vi "HEWH Sampled Data String.vi"(8 "error in (no error)":errorcluster, 11 "UEF Calculated Values Output in":T1 {"Data Indexes"."15 sec after Draw Index" format="%#.2f"; "Data Indexes"."15 sec after Draw Timestamp" format="%#.2f"; "Data Indexes"."Test Start Timestamp" format="%.2f"; "Data Indexes"."Test End Timestamp" format="%.2f"; "Data Indexes"."T0 Timestamp" format="%.2f"; "Data Indexes"."Tsf Timestamp" format="%.2f"; "Data Indexes"."Tsu0 Timestamp" format="%.2f"; "Data Indexes"."Tmax1 Timestamp" format="%.2f"; "Data Indexes"."Draw Index Timestamp" format="%#.2f"; "Data Indexes"."Non-Draw Timestamp" format="%#.2f"; "Data Indexes"."Heating Timestamp" format="%#.2f"; "Data Indexes"."Start Energy (BTU-Gas)" format="%.6f"; "Data Indexes"."Start Watt Hours" format="%.6f"; "Static Data"."V - Volume of Wh (True)" format="%.5f"; "Static Data"."T-Ambinet Nominal (°F)" format="%.5f"; "Static Data"."T-Inlet Setpoint (°F)" format="%.5f"; "Static Data"."T-Wh Setpoint (°F)" format="%.5f"; "Sampled Data"."Qe (Wh)" format="%.5f"; "Sampled Data"."Tau stby2 (hr)" format="%.5f"; "Sampled Data"."Tastby2 (°F)" format="%.5f"; "Sampled Data"."Qf (BTU)" format="%.5f"; "Sampled Data"."Qe (BTU)" format="%.5f"; "Sampled Data"."Tmax1 (°F)" format="%.5f"; "Sampled Data"."T0 (°F)" format="%.5f"; "Sampled Data"."Qr (BTU)" format="%.5f"; "Sampled Data"."T 24(°F)" format="%.5f"; "Sampled Data"."T astby(°F)" format="%.5f"; "Sampled Data"."T tstby(°F)" format="%.5f"; "Sampled Data"."T su0(°F)" format="%.5f"; "Sampled Data"."T suf(°F)" format="%.5f"; "Sampled Data"."Tau stby_1 (hr)" format="%.5f"; "Sampled Data"."Qsuf (BTU)" format="%.5f"; "Sampled Data"."Qsu0 (BTU)" format="%.5f"; "Calculated Values"."Draw Bonus Volume (gal)" format="%.6f"; "Calculated Values"."Adjustment Factor" format="%.6f"; "Calculated Values"."T*avg_del(n-1)" format="%.6f"; "Calculated Values"."T*min(n-1)" format="%.6f"; "Calculated Values"."T*avg_del(n)" format="%.6f"; "Calculated Values"."Vn" format="%.6f"; "Calculated Values"."Qdm (BTU)" format="%.6f"; "Calculated Values"."QHWD (BTU)" format="%.6f"; "Calculated Values"."QHW (BTU)" format="%.6f"; "Calculated Values"."UEF" format="%.6f"; "Calculated Values"."QHW67 (BTU)" format="%.6f"; "Calculated Values"."Qda (BTU)" format="%.6f"; "Calculated Values"."Qd (BTU)" format="%.6f"; "Calculated Values"."Q (BTU)" format="%.6f"; "Calculated Values"."UA (BTU/(hr*F))" format="%.6f"; "Calculated Values"."Qhr (BTU/hr)" format="%.6f"; "Calculated Values"."Qstby (BTU)" format="%.6f"; "Calculated Values"."nu_r" format="%.6f"; "Calculated Values"."CpUEF (BTU/(lb*F))" format="%.6f"; "Calculated Values"."rho_nu (lb/gal)" format="%.6f"; "Calculated Values"."V1- Vol (Gal)" format="%.6f"; "Calculated Values"."M cluster mass removed (lb)" format="%.6f"; "Calculated Values"."Cp theoretical (BTU/(lbm °F))" format="%.6f"; "Calculated Values"."Tin1 - Mean Inlet 1st Cluster (°F)" format="%.6f"; "Calculated Values"."Tdel1-Mean Outlet 1st Cluster(°F)" format="%.6f"; "Calculated Values"."Cp 24 (BTU/(lb*F))" format="%.6f"; "Calculated Values"."Cp standby (BTU/(lb*F))" format="%.6f"; "Calculated Values"."Cp2 (BTU/(lb*F))" format="%.6f"; "Calculated Values"."Cp1 (BTU/(lb*F))" format="%.6f"; "Calculated Values"."rho 24 (lb/gal)" format="%.6f"; "Calculated Values"."rho standby (lb/gal)" format="%.6f"; "Calculated Values"."rho 2 (lb/gal)" format="%.6f"; "Calculated Values"."Density of cold water All (lbm/gal)" format="%#.3g"; "Calculated Values"."CpHW (BTU/(lbm °F))" format="%#.3g"; "Calculated Values"."Density of hot water All (lbm/gal)" format="%#.3g"; "Calculated Values"."Mass of water All (lbm)" format="%#.3f"}) -> (0 "error out":errorcluster, 3 "UEF Calculated Values Output out":T1 {"Data Indexes"."15 sec after Draw Index" format="%#.2f"; "Data Indexes"."15 sec after Draw Timestamp" format="%#.2f"; "Data Indexes"."Test Start Timestamp" format="%.2f"; "Data Indexes"."Test End Timestamp" format="%.2f"; "Data Indexes"."T0 Timestamp" format="%.2f"; "Data Indexes"."Tsf Timestamp" format="%.2f"; "Data Indexes"."Tsu0 Timestamp" format="%.2f"; "Data Indexes"."Tmax1 Timestamp" format="%.2f"; "Data Indexes"."Draw Index Timestamp" format="%#.2f"; "Data Indexes"."Non-Draw Timestamp" format="%#.2f"; "Data Indexes"."Heating Timestamp" format="%#.2f"; "Data Indexes"."Start Energy (BTU-Gas)" format="%.6f"; "Data Indexes"."Start Watt Hours" format="%.6f"; "Static Data"."V - Volume of Wh (True)" format="%.5f"; "Static Data"."T-Ambinet Nominal (°F)" format="%.5f"; "Static Data"."T-Inlet Setpoint (°F)" format="%.5f"; "Static Data"."T-Wh Setpoint (°F)" format="%.5f"; "Sampled Data"."Qe (Wh)" format="%.5f"; "Sampled Data"."Tau stby2 (hr)" format="%.5f"; "Sampled Data"."Tastby2 (°F)" format="%.5f"; "Sampled Data"."Qf (BTU)" format="%.5f"; "Sampled Data"."Qe (BTU)" format="%.5f"; "Sampled Data"."Tmax1 (°F)" format="%.5f"; "Sampled Data"."T0 (°F)" format="%.5f"; "Sampled Data"."Qr (BTU)" format="%.5f"; "Sampled Data"."T 24(°F)" format="%.5f"; "Sampled Data"."T astby(°F)" format="%.5f"; "Sampled Data"."T tstby(°F)" format="%.5f"; "Sampled Data"."T su0(°F)" format="%.5f"; "Sampled Data"."T suf(°F)" format="%.5f"; "Sampled Data"."Tau stby_1 (hr)" format="%.5f"; "Sampled Data"."Qsuf (BTU)" format="%.5f"; "Sampled Data"."Qsu0 (BTU)" format="%.5f"; "Calculated Values"."Draw Bonus Volume (gal)" format="%.6f"; "Calculated Values"."Adjustment Factor" format="%.6f"; "Calculated Values"."T*avg_del(n-1)" format="%.6f"; "Calculated Values"."T*min(n-1)" format="%.6f"; "Calculated Values"."T*avg_del(n)" format="%.6f"; "Calculated Values"."Vn" format="%.6f"; "Calculated Values"."Qdm (BTU)" format="%.6f"; "Calculated Values"."QHWD (BTU)" format="%.6f"; "Calculated Values"."QHW (BTU)" format="%.6f"; "Calculated Values"."UEF" format="%.6f"; "Calculated Values"."QHW67 (BTU)" format="%.6f"; "Calculated Values"."Qda (BTU)" format="%.6f"; "Calculated Values"."Qd (BTU)" format="%.6f"; "Calculated Values"."Q (BTU)" format="%.6f"; "Calculated Values"."UA (BTU/(hr*F))" format="%.6f"; "Calculated Values"."Qhr (BTU/hr)" format="%.6f"; "Calculated Values"."Qstby (BTU)" format="%.6f"; "Calculated Values"."nu_r" format="%.6f"; "Calculated Values"."CpUEF (BTU/(lb*F))" format="%.6f"; "Calculated Values"."rho_nu (lb/gal)" format="%.6f"; "Calculated Values"."V1- Vol (Gal)" format="%.6f"; "Calculated Values"."M cluster mass removed (lb)" format="%.6f"; "Calculated Values"."Cp theoretical (BTU/(lbm °F))" format="%.6f"; "Calculated Values"."Tin1 - Mean Inlet 1st Cluster (°F)" format="%.6f"; "Calculated Values"."Tdel1-Mean Outlet 1st Cluster(°F)" format="%.6f"; "Calculated Values"."Cp 24 (BTU/(lb*F))" format="%.6f"; "Calculated Values"."Cp standby (BTU/(lb*F))" format="%.6f"; "Calculated Values"."Cp2 (BTU/(lb*F))" format="%.6f"; "Calculated Values"."Cp1 (BTU/(lb*F))" format="%.6f"; "Calculated Values"."rho 24 (lb/gal)" format="%.6f"; "Calculated Values"."rho standby (lb/gal)" format="%.6f"; "Calculated Values"."rho 2 (lb/gal)" format="%.6f"; "Calculated Values"."Density of cold water All (lbm/gal)" format="%#.3g"; "Calculated Values"."CpHW (BTU/(lbm °F))" format="%#.3g"; "Calculated Values"."Density of hot water All (lbm/gal)" format="%#.3g"; "Calculated Values"."Mass of water All (lbm)" format="%#.3f"})   [LabVIEW 2023]
uses:
  Type Definitions/UEF Constants.ctl
  Type Definitions/HEWH Draw Stats.ctl
  Type Definitions/HEWH FHR Draw Type.ctl
  Type Definitions/FHR Bins.ctl
  Type Definitions/HEWH Meter Type.ctl
panel:
  # "FHR"
  # "FHR"
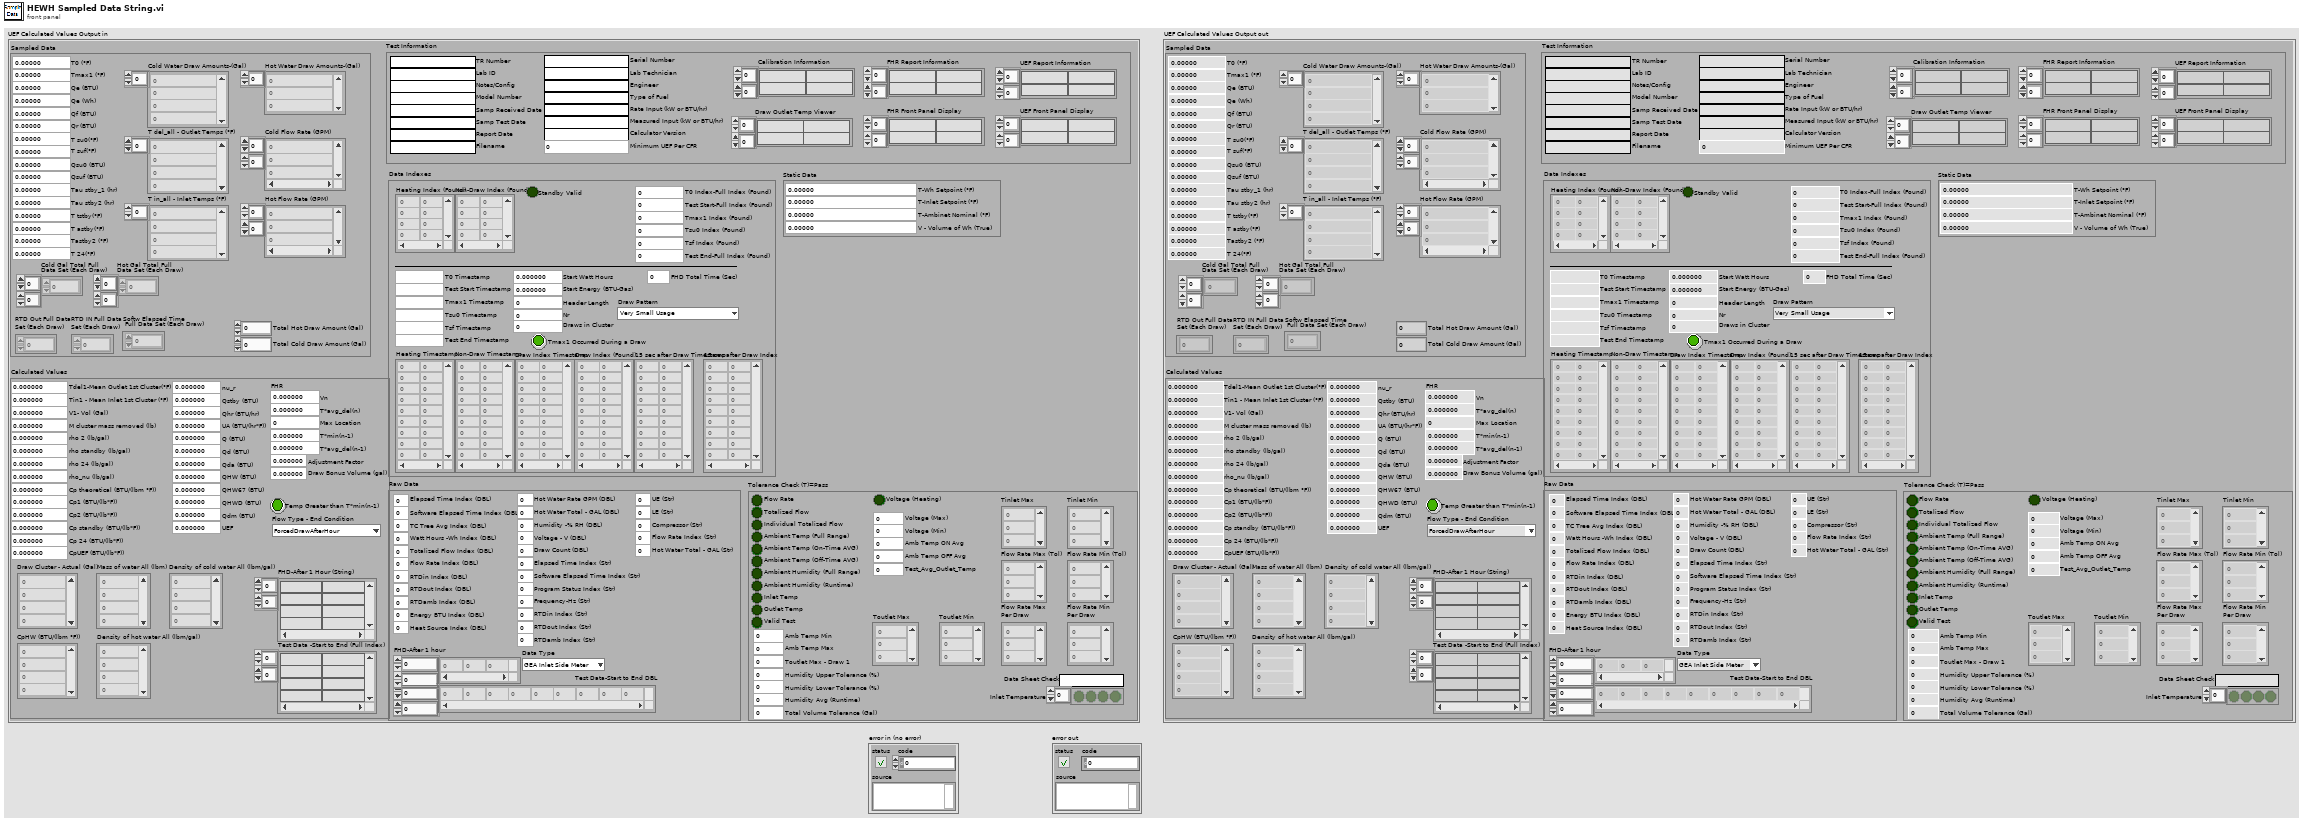
[diagram p1: front panel]
types:
  T1 = typedef "UEF Constants.ctl" = cluster{"Calculated Values":T2, "Sampled Data":cluster{"Cold Water Draw Amounts-(Gal)":dbl[], "T del_all - Outlet Temps (°F)":dbl[], "T in_all - Inlet Temps (°F)":dbl[], "Qsu0 (BTU)":dbl, "Qsuf (BTU)":dbl, "Tau stby_1 (hr)":dbl, "T suf(°F)":dbl, "T su0(°F)":dbl, "T tstby(°F)":dbl, "T astby(°F)":dbl, "T 24(°F)":dbl, "Qr (BTU)":dbl, "T0 (°F)":dbl, "Tmax1 (°F)":dbl, "Qe (BTU)":dbl, "Qf (BTU)":dbl, "Tastby2 (°F)":dbl, "RTD Out Full Data\nSet (Each Draw)":dbl[][], "RTD IN Full Data\nSet (Each Draw)":dbl[][], "Tau stby2 (hr)":dbl, "Hot Water Draw Amounts-(Gal)":dbl[], "Cold Flow Rate (GPM)":dbl[][], "Hot Flow Rate (GPM)":dbl[][], "Softw Elapsed Time\n Full Data Set (Each Draw)":dbl[][], "Cold Gal Total Full\nData Set (Each Draw)":dbl[][], "Total Hot Draw Amount (Gal) ":dbl, "Total Cold Draw Amount (Gal)":dbl, "Qe (Wh)":dbl, "Hot Gal Total Full\nData Set (Each Draw)":dbl[][]}, "Static Data":cluster{"T-Wh Setpoint (°F)":dbl, "T-Inlet Setpoint (°F)":dbl, "T-Ambinet Nominal (°F)":dbl, "V - Volume of Wh (True)":dbl}, "Data Indexes":cluster{"Test Start-Full Index (Found)":i32, "Header Length":i32, "Draw Index (Found)":i32[][], "Nr":i32, "Start Watt Hours":dbl, "Tsu0 Index (Found)":i32, "Tsf Index (Found)":i32, "Start Energy (BTU-Gas)":dbl, "Draws in Cluster":i32, "T0 Index-Full Index (Found)":i32, "Non-Draw Index (Found)":i32[][], "Tmax1 Index (Found)":i32, "Test End-Full Index (Found)":i32, "Heating Index (Found)":i32[][], "Heating Timestamp":dbl[][], "Non-Draw Timestamp":dbl[][], "Draw Index Timestamp":dbl[][], "Tmax1 Timestamp":dbl, "Tsu0 Timestamp":dbl, "Tsf Timestamp":dbl, "T0 Timestamp":dbl, "Test End Timestamp":dbl, "Test Start Timestamp":dbl, "15 sec after Draw Timestamp":dbl[][], "15 sec after Draw Index":dbl[][], "Tmax1 Occurred During a Draw":bool, "FHD Total Time (Sec)":dbl, "Draw Pattern":T4, "Standby Valid":bool}, "Raw Data":cluster{"Elapsed Time Index (DBL)":i32, "Software Elapsed Time Index (DBL)":i32, "TC Tree Avg Index (DBL)":i32, "Watt Hours -Wh Index (DBL)":i32, "Energy BTU Index (DBL)":i32, "Totalized Flow Index (DBL)":i32, "Flow Rate Index (DBL)":i32, "Program Status Index (Str)":i32, "RTDin Index (DBL)":i32, "RTDout Index (DBL)":i32, "RTDamb Index (DBL)":i32, "Test Data-Start to End DBL":dbl[][], "Data Type":T5, "Heat Source Index (DBL)":i32, "Hot Water Rate GPM (DBL)":i32, "Hot Water Total - GAL (DBL)":i32, "FHD-After 1 hour":dbl[][], "Humidity -% RH (DBL)":i32, "Voltage - V (DBL)":i32, "Draw Count (DBL)":i32, "Elapsed Time Index (Str)":i32, "Software Elapsed Time Index (Str)":i32, "Frequency-Hz (Str)":i32, "RTDin Index (Str)":i32, "RTDout Index (Str)":i32, "RTDamb Index (Str)":i32, "UE (Str)":i32, "LE (Str)":i32, "Compressor (Str)":i32, "Flow Rate Index (Str)":i32, "Hot Water Total - GAL (Str)":i32}, "Tolerance Check (T)=Pass":cluster{"Flow Rate":bool, "Totalized Flow":bool, "Ambient Temp (Full Range)":bool, "Ambient Humidity (Full Range)":bool, "Inlet Temp":bool, "Outlet Temp":bool, "Valid Test":bool, "Individual Totalized Flow":bool, "Data Sheet Check":string, "Inlet Temperature":bool[], "Tinlet Max":dbl[], "Tinlet Min":dbl[], "Flow Rate Max (Tol)":dbl[], "Flow Rate Min (Tol)":dbl[], "Amb Temp Max":dbl, "Amb Temp Min":dbl, "Toutlet Max - Draw 1":dbl, "Humidity Upper Tolerance (%)":dbl, "Total Volume Tolerance (Gal)":dbl, "Humidity Lower Tolerance (%)":dbl, "Flow Rate Max\nPer Draw":dbl[], "Flow Rate Min\nPer Draw":dbl[], "Ambient Humidity (Runtime)":bool, "Humidity Avg (Runtime)":dbl, "Ambient Temp (On-Time AVG)":bool, "Ambient Temp (Off-Time AVG)":bool, "Amb Temp OFF Avg":dbl, "Amb Temp ON Avg":dbl, "Voltage (Heating)":bool, "Voltage (Min)":dbl, "Voltage (Max)":dbl, "Toutlet Max":dbl[], "Toutlet Min":dbl[], "Test_Avg_Outlet_Temp":dbl}, "Test Information":cluster{"TR Number":string, "Lab ID":string, "Notes/Config":string, "Model Number":string, "Serial Number":string, "Lab Technician":string, "Engineer":string, "Type of Fuel":string, "Samp Received Date":string, "Samp Test Date":string, "Report Date":string, "Rate Input (kW or BTU/hr)":string, "Measured Input (kW or BTU/hr)":string, "Filename":string, "Calibration Information":string[][], "Calculator Version":string, "Minimum UEF Per CFR":dbl, "UEF Report Information":string[][], "FHR Report Information":string[][], "FHR Front Panel Display":string[][], "UEF Front Panel Display":string[][], "Draw Outlet Temp Viewer":string[][]}}
  T2 = typedef "HEWH Draw Stats.ctl" = cluster{"Draw Cluster - Actual (Gal)":dbl[], "Mass of water All (lbm)":dbl[], "Density of hot water All (lbm/gal)":dbl[], "CpHW (BTU/(lbm °F))":dbl[], "rho 2 (lb/gal)":dbl, "rho standby (lb/gal)":dbl, "rho 24 (lb/gal)":dbl, "Cp1 (BTU/(lb*F))":dbl, "Cp2 (BTU/(lb*F))":dbl, "Cp standby (BTU/(lb*F))":dbl, "Cp 24 (BTU/(lb*F))":dbl, "nu_r":dbl, "Qstby (BTU)":dbl, "Qhr (BTU/hr)":dbl, "UA (BTU/(hr*F))":dbl, "Q (BTU)":dbl, "Qd (BTU)":dbl, "Qda (BTU)":dbl, "QHW67 (BTU)":dbl, "UEF":dbl, "Tdel1-Mean Outlet 1st Cluster(°F)":dbl, "Tin1 - Mean Inlet 1st Cluster (°F)":dbl, "Cp theoretical (BTU/(lbm °F))":dbl, "M cluster mass removed (lb)":dbl, "V1- Vol (Gal)":dbl, "Test Data -Start to End (Full Index)":string[][], "rho_nu (lb/gal)":dbl, "Density of cold water All (lbm/gal)":dbl[], "CpUEF (BTU/(lb*F))":dbl, "QHW (BTU)":dbl, "QHWD (BTU)":dbl, "Qdm (BTU)":dbl, "FHD-After 1 Hour (String)":string[][], "Vn":dbl, "T*avg_del(n)":dbl, "Max Location":i32, "T*min(n-1)":dbl, "T*avg_del(n-1)":dbl, "Temp Greater than T*min(n-1)":bool, "Adjustment Factor":dbl, "Draw Bonus Volume (gal)":dbl, "Flow Type - End Condition":T3}
  T3 = typedef "HEWH FHR Draw Type.ctl" = enum16{"ForcedDrawAfterHour", "HeatingCutoffBeforeHour"}
  T4 = typedef "FHR Bins.ctl" = enum16{"Very Small Usage", "Low Usage", "Medium Usage", "High Usage", "Undefined"}
  T5 = typedef "HEWH Meter Type.ctl" = enum16{"GEA Inlet Side Meter", "GEA Outlet Side Meter", "CSA Inlet Side Meter"}
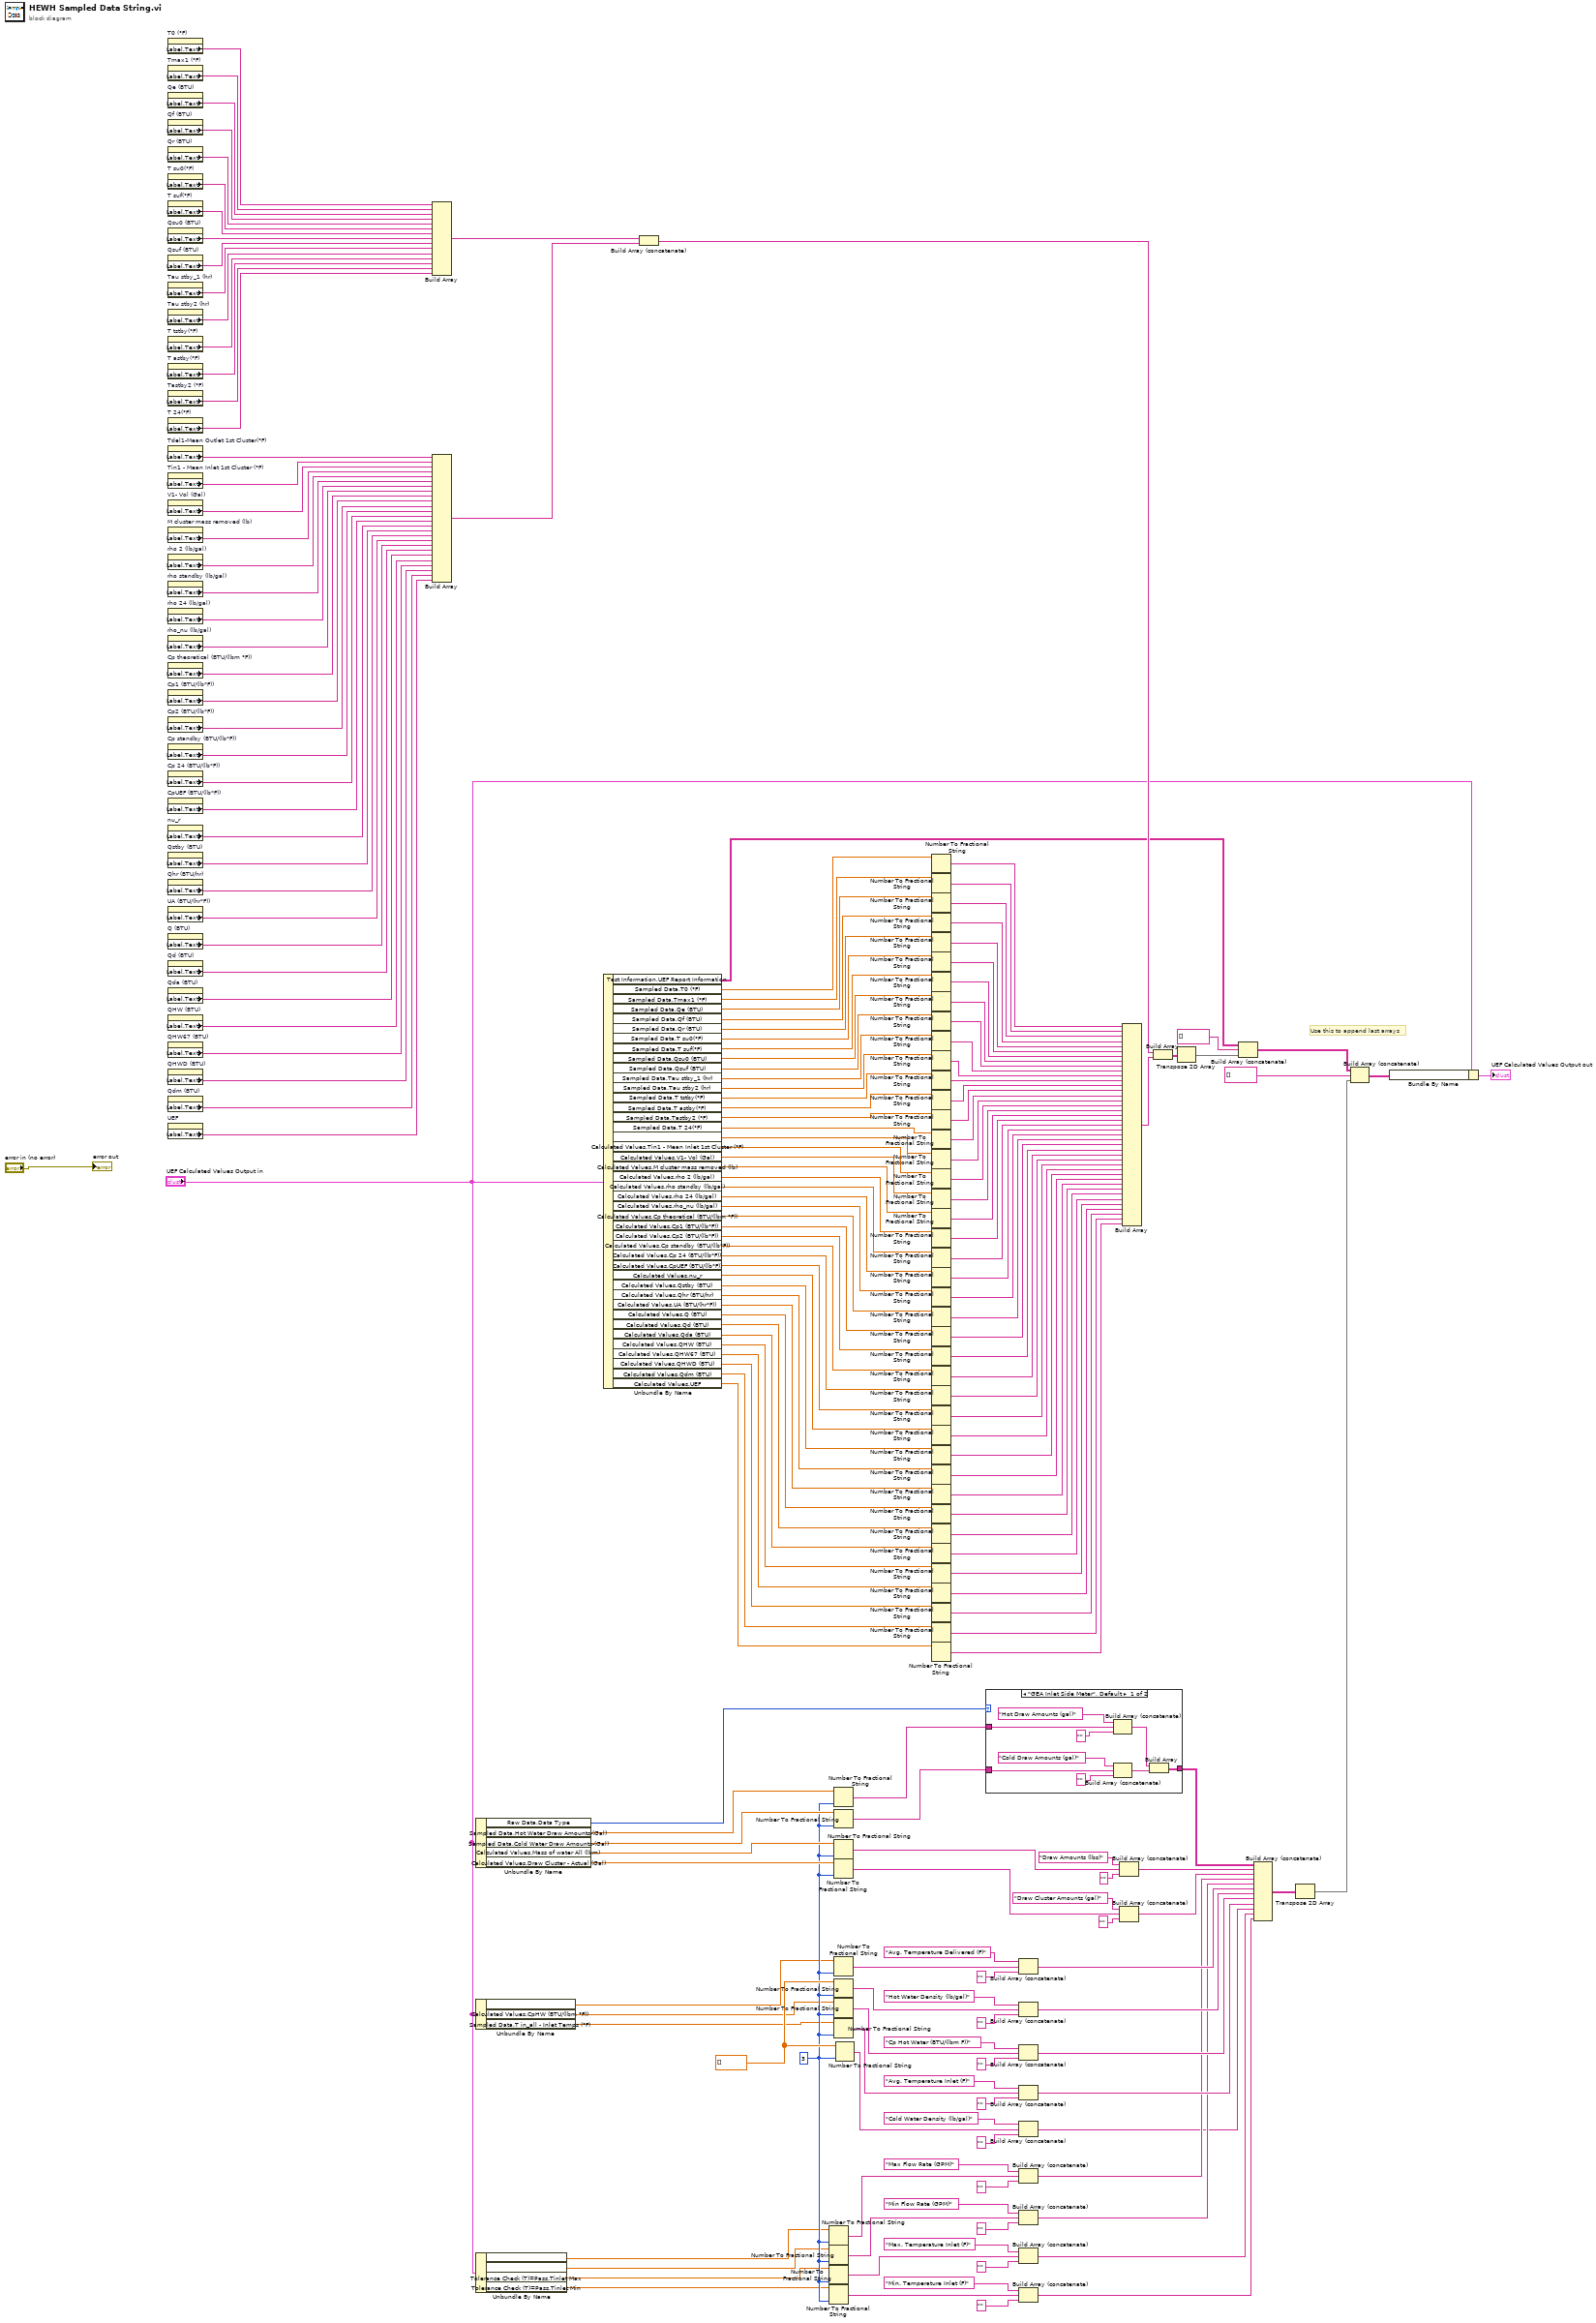
[diagram p0: block diagram]
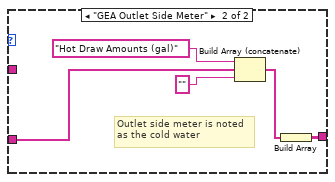
[diagram p2: hidden frame]
diagram:
  w64 = dbl[] []
  w22 = i16 3 ("precision (6)")
  # "Use this to append last arrays"
  n1 = property on="T0 (°F)" class="DigNum (strict)"() -> ("Label.Text"=w170:string)  [unwired: 2 in, 2 out]
  n2 = property on="Tmax1 (°F)" class="DigNum (strict)"() -> ("Label.Text"=w169:string)  [unwired: 2 in, 2 out]
  n3 = property on="Qe (BTU)" class="DigNum (strict)"() -> ("Label.Text"=w168:string)  [unwired: 2 in, 2 out]
  n4 = property on="Qf (BTU)" class="DigNum (strict)"() -> ("Label.Text"=w167:string)  [unwired: 2 in, 2 out]
  n5 = property on="Qr (BTU)" class="DigNum (strict)"() -> ("Label.Text"=w166:string)  [unwired: 2 in, 2 out]
  n6 = property on="T su0(°F)" class="DigNum (strict)"() -> ("Label.Text"=w165:string)  [unwired: 2 in, 2 out]
  n7 = property on="T suf(°F)" class="DigNum (strict)"() -> ("Label.Text"=w164:string)  [unwired: 2 in, 2 out]
  n8 = property on="Qsu0 (BTU)" class="DigNum (strict)"() -> ("Label.Text"=w163:string)  [unwired: 2 in, 2 out]
  n9 = property on="Qsuf (BTU)" class="DigNum (strict)"() -> ("Label.Text"=w162:string)  [unwired: 2 in, 2 out]
  n10 = property on="Tau stby_1 (hr)" class="DigNum (strict)"() -> ("Label.Text"=w161:string)  [unwired: 2 in, 2 out]
  n11 = property on="Tau stby2 (hr)" class="DigNum (strict)"() -> ("Label.Text"=w160:string)  [unwired: 2 in, 2 out]
  n12 = property on="T tstby(°F)" class="DigNum (strict)"() -> ("Label.Text"=w159:string)  [unwired: 2 in, 2 out]
  n13 = property on="T astby(°F)" class="DigNum (strict)"() -> ("Label.Text"=w158:string)  [unwired: 2 in, 2 out]
  n14 = property on="Tastby2 (°F)" class="DigNum (strict)"() -> ("Label.Text"=w157:string)  [unwired: 2 in, 2 out]
  n15 = property on="T 24(°F)" class="DigNum (strict)"() -> ("Label.Text"=w156:string)  [unwired: 2 in, 2 out]
  n16 = property on="Tdel1-Mean Outlet 1st Cluster(°F)" class="DigNum (strict)"() -> ("Label.Text"=w96:string)  [unwired: 2 in, 2 out]
  n17 = property on="Tin1 - Mean Inlet 1st Cluster (°F)" class="DigNum (strict)"() -> ("Label.Text"=w95:string)  [unwired: 2 in, 2 out]
  n18 = property on="V1- Vol (Gal)" class="DigNum (strict)"() -> ("Label.Text"=w94:string)  [unwired: 2 in, 2 out]
  n19 = property on="M cluster mass removed (lb)" class="DigNum (strict)"() -> ("Label.Text"=w93:string)  [unwired: 2 in, 2 out]
  n20 = property on="rho 2 (lb/gal)" class="DigNum (strict)"() -> ("Label.Text"=w92:string)  [unwired: 2 in, 2 out]
  n21 = property on="rho standby (lb/gal)" class="DigNum (strict)"() -> ("Label.Text"=w91:string)  [unwired: 2 in, 2 out]
  n22 = property on="rho 24 (lb/gal)" class="DigNum (strict)"() -> ("Label.Text"=w90:string)  [unwired: 2 in, 2 out]
  n23 = property on="rho_nu (lb/gal)" class="DigNum (strict)"() -> ("Label.Text"=w89:string)  [unwired: 2 in, 2 out]
  n24 = property on="Cp theoretical (BTU/(lbm °F))" class="DigNum (strict)"() -> ("Label.Text"=w88:string)  [unwired: 2 in, 2 out]
  n25 = property on="Cp1 (BTU/(lb*F))" class="DigNum (strict)"() -> ("Label.Text"=w87:string)  [unwired: 2 in, 2 out]
  n26 = property on="Cp2 (BTU/(lb*F))" class="DigNum (strict)"() -> ("Label.Text"=w86:string)  [unwired: 2 in, 2 out]
  n27 = property on="Cp standby (BTU/(lb*F))" class="DigNum (strict)"() -> ("Label.Text"=w85:string)  [unwired: 2 in, 2 out]
  n28 = property on="Cp 24 (BTU/(lb*F))" class="DigNum (strict)"() -> ("Label.Text"=w84:string)  [unwired: 2 in, 2 out]
  n29 = property on="CpUEF (BTU/(lb*F))" class="DigNum (strict)"() -> ("Label.Text"=w83:string)  [unwired: 2 in, 2 out]
  n30 = property on="nu_r" class="DigNum (strict)"() -> ("Label.Text"=w82:string)  [unwired: 2 in, 2 out]
  n31 = property on="Qstby (BTU)" class="DigNum (strict)"() -> ("Label.Text"=w81:string)  [unwired: 2 in, 2 out]
  n32 = property on="Qhr (BTU/hr)" class="DigNum (strict)"() -> ("Label.Text"=w80:string)  [unwired: 2 in, 2 out]
  n33 = property on="UA (BTU/(hr*F))" class="DigNum (strict)"() -> ("Label.Text"=w79:string)  [unwired: 2 in, 2 out]
  n34 = property on="Q (BTU)" class="DigNum (strict)"() -> ("Label.Text"=w78:string)  [unwired: 2 in, 2 out]
  n35 = property on="Qd (BTU)" class="DigNum (strict)"() -> ("Label.Text"=w77:string)  [unwired: 2 in, 2 out]
  n36 = property on="Qda (BTU)" class="DigNum (strict)"() -> ("Label.Text"=w76:string)  [unwired: 2 in, 2 out]
  n37 = property on="QHW (BTU)" class="DigNum (strict)"() -> ("Label.Text"=w75:string)  [unwired: 2 in, 2 out]
  n38 = property on="QHW67 (BTU)" class="DigNum (strict)"() -> ("Label.Text"=w74:string)  [unwired: 2 in, 2 out]
  n39 = property on="QHWD (BTU)" class="DigNum (strict)"() -> ("Label.Text"=w73:string)  [unwired: 2 in, 2 out]
  n40 = property on="Qdm (BTU)" class="DigNum (strict)"() -> ("Label.Text"=w72:string)  [unwired: 2 in, 2 out]
  n41 = property on="UEF" class="DigNum (strict)"() -> ("Label.Text"=w71:string)  [unwired: 2 in, 2 out]
  n42 = Build Array(w170, w169, w168, w167, w166, w165, w164, w163, w162, w161, w160, w159, w158, w157, w156) -> (w70:string[])
  n43 = Build Array(w96, w95, w94, w93, w92, w91, w90, w89, w88, w87, w86, w85, w84, w83, w82, w81, w80, w79, w78, w77, w76, w75, w74, w73, w72, w71) -> (w69:string[])
  n44 = Unbundle By Name("UEF Calculated Values Output in") -> ("Raw Data.Data Type"=w33:T5, "Sampled Data.Hot Water Draw Amounts-(Gal)"=w35:dbl[], "Sampled Data.Cold Water Draw Amounts-(Gal)"=w63:dbl[], "Calculated Values.Mass of water All (lbm)"=w61:dbl[], "Calculated Values.Draw Cluster - Actual (Gal)"=w62:dbl[])
  n45 = Unbundle By Name("UEF Calculated Values Output in") -> ("Sampled Data.T del_all - Outlet Temps (°F)"=w16:dbl[], "Calculated Values.CpHW (BTU/(lbm °F))"=w15:dbl[], "Sampled Data.T in_all - Inlet Temps (°F)"=w14:dbl[])
  n46 = Unbundle By Name("UEF Calculated Values Output in") -> ("Tolerance Check (T)=Pass.Flow Rate Max\nPer Draw"=w10:dbl[], "Tolerance Check (T)=Pass.Flow Rate Min\nPer Draw"=w9:dbl[], "Tolerance Check (T)=Pass.Tinlet Max"=w8:dbl[], "Tolerance Check (T)=Pass.Tinlet Min"=w7:dbl[])
  n47 = Unbundle By Name("UEF Calculated Values Output in") -> ("Test Information.UEF Report Information"=w67:string[][], "Sampled Data.T0 (°F)"=w200:dbl, "Sampled Data.Tmax1 (°F)"=w199:dbl, "Sampled Data.Qe (BTU)"=w198:dbl, "Sampled Data.Qf (BTU)"=w197:dbl, "Sampled Data.Qr (BTU)"=w196:dbl, "Sampled Data.T su0(°F)"=w195:dbl, "Sampled Data.T suf(°F)"=w194:dbl, "Sampled Data.Qsu0 (BTU)"=w193:dbl, "Sampled Data.Qsuf (BTU)"=w192:dbl, "Sampled Data.Tau stby_1 (hr)"=w191:dbl, "Sampled Data.Tau stby2 (hr)"=w190:dbl, "Sampled Data.T tstby(°F)"=w189:dbl, "Sampled Data.T astby(°F)"=w188:dbl, "Sampled Data.Tastby2 (°F)"=w187:dbl, "Sampled Data.T 24(°F)"=w186:dbl, "Calculated Values.Tdel1-Mean Outlet 1st Cluster(°F)"=w148:dbl, "Calculated Values.Tin1 - Mean Inlet 1st Cluster (°F)"=w147:dbl, "Calculated Values.V1- Vol (Gal)"=w146:dbl, "Calculated Values.M cluster mass removed (lb)"=w145:dbl, "Calculated Values.rho 2 (lb/gal)"=w144:dbl, "Calculated Values.rho standby (lb/gal)"=w143:dbl, "Calculated Values.rho 24 (lb/gal)"=w142:dbl, "Calculated Values.rho_nu (lb/gal)"=w141:dbl, "Calculated Values.Cp theoretical (BTU/(lbm °F))"=w140:dbl, "Calculated Values.Cp1 (BTU/(lb*F))"=w139:dbl, "Calculated Values.Cp2 (BTU/(lb*F))"=w138:dbl, "Calculated Values.Cp standby (BTU/(lb*F))"=w137:dbl, "Calculated Values.Cp 24 (BTU/(lb*F))"=w136:dbl, "Calculated Values.CpUEF (BTU/(lb*F))"=w135:dbl, "Calculated Values.nu_r"=w134:dbl, "Calculated Values.Qstby (BTU)"=w133:dbl, "Calculated Values.Qhr (BTU/hr)"=w132:dbl, "Calculated Values.UA (BTU/(hr*F))"=w131:dbl, "Calculated Values.Q (BTU)"=w130:dbl, "Calculated Values.Qd (BTU)"=w129:dbl, "Calculated Values.Qda (BTU)"=w128:dbl, "Calculated Values.QHW (BTU)"=w127:dbl, "Calculated Values.QHW67 (BTU)"=w126:dbl, "Calculated Values.QHWD (BTU)"=w125:dbl, "Calculated Values.Qdm (BTU)"=w124:dbl, "Calculated Values.UEF"=w123:dbl)
  n48 = Build Array (concatenate)(w70, w69) -> (w68:string[])
  n49 = Number To Fractional String(number=w10, precision (6)=w22) -> (F-format string=w21:string[])  [unwired: 2 in]
  n50 = Number To Fractional String(number=w9, precision (6)=w22) -> (F-format string=w20:string[])  [unwired: 2 in]
  n51 = Number To Fractional String(number=w8, precision (6)=w22) -> (F-format string=w28:string[])  [unwired: 2 in]
  n52 = Number To Fractional String(number=w7, precision (6)=w22) -> (F-format string=w27:string[])  [unwired: 2 in]
  n53 = Number To Fractional String(number=w35, precision (6)=w22) -> (F-format string=w34:string[])  [unwired: 2 in]
  n54 = Number To Fractional String(number=w63, precision (6)=w22) -> (F-format string=w60:string[])  [unwired: 2 in]
  n55 = Number To Fractional String(number=w61, precision (6)=w22) -> (F-format string=w59:string[])  [unwired: 2 in]
  n56 = Number To Fractional String(number=w62, precision (6)=w22) -> (F-format string=w55:string[])  [unwired: 2 in]
  n57 = Number To Fractional String(number=w16, precision (6)=w22) -> (F-format string=w54:string[])  [unwired: 2 in]
  n58 = Number To Fractional String(number=w64, precision (6)=w22) -> (F-format string=w53:string[])  [unwired: 2 in]
  n59 = Number To Fractional String(number=w15, precision (6)=w22) -> (F-format string=w52:string[])  [unwired: 2 in]
  n60 = Number To Fractional String(number=w14, precision (6)=w22) -> (F-format string=w51:string[])  [unwired: 2 in]
  n61 = Number To Fractional String(number=w64, precision (6)=w22) -> (F-format string=w50:string[])  [unwired: 2 in]
  n62 = Number To Fractional String(number=w200) -> (F-format string=w185:string)  [unwired: 3 in]
  n63 = Number To Fractional String(number=w199) -> (F-format string=w184:string)  [unwired: 3 in]
  n64 = Number To Fractional String(number=w198) -> (F-format string=w183:string)  [unwired: 3 in]
  n65 = Number To Fractional String(number=w197) -> (F-format string=w182:string)  [unwired: 3 in]
  n66 = Number To Fractional String(number=w196) -> (F-format string=w181:string)  [unwired: 3 in]
  n67 = Number To Fractional String(number=w195) -> (F-format string=w180:string)  [unwired: 3 in]
  n68 = Number To Fractional String(number=w194) -> (F-format string=w179:string)  [unwired: 3 in]
  n69 = Number To Fractional String(number=w193) -> (F-format string=w178:string)  [unwired: 3 in]
  n70 = Number To Fractional String(number=w192) -> (F-format string=w177:string)  [unwired: 3 in]
  n71 = Number To Fractional String(number=w191) -> (F-format string=w176:string)  [unwired: 3 in]
  n72 = Number To Fractional String(number=w190) -> (F-format string=w175:string)  [unwired: 3 in]
  n73 = Number To Fractional String(number=w189) -> (F-format string=w174:string)  [unwired: 3 in]
  n74 = Number To Fractional String(number=w188) -> (F-format string=w173:string)  [unwired: 3 in]
  n75 = Number To Fractional String(number=w187) -> (F-format string=w172:string)  [unwired: 3 in]
  n76 = Number To Fractional String(number=w186) -> (F-format string=w171:string)  [unwired: 3 in]
  n77 = Number To Fractional String(number=w148) -> (F-format string=w122:string)  [unwired: 3 in]
  n78 = Number To Fractional String(number=w147) -> (F-format string=w121:string)  [unwired: 3 in]
  n79 = Number To Fractional String(number=w146) -> (F-format string=w120:string)  [unwired: 3 in]
  n80 = Number To Fractional String(number=w145) -> (F-format string=w119:string)  [unwired: 3 in]
  n81 = Number To Fractional String(number=w144) -> (F-format string=w118:string)  [unwired: 3 in]
  n82 = Number To Fractional String(number=w143) -> (F-format string=w117:string)  [unwired: 3 in]
  n83 = Number To Fractional String(number=w142) -> (F-format string=w116:string)  [unwired: 3 in]
  n84 = Number To Fractional String(number=w141) -> (F-format string=w115:string)  [unwired: 3 in]
  n85 = Number To Fractional String(number=w140) -> (F-format string=w114:string)  [unwired: 3 in]
  n86 = Number To Fractional String(number=w139) -> (F-format string=w113:string)  [unwired: 3 in]
  n87 = Number To Fractional String(number=w138) -> (F-format string=w112:string)  [unwired: 3 in]
  n88 = Number To Fractional String(number=w137) -> (F-format string=w111:string)  [unwired: 3 in]
  n89 = Number To Fractional String(number=w136) -> (F-format string=w110:string)  [unwired: 3 in]
  n90 = Number To Fractional String(number=w135) -> (F-format string=w109:string)  [unwired: 3 in]
  n91 = Number To Fractional String(number=w134) -> (F-format string=w108:string)  [unwired: 3 in]
  n92 = Number To Fractional String(number=w133) -> (F-format string=w107:string)  [unwired: 3 in]
  n93 = Number To Fractional String(number=w132) -> (F-format string=w106:string)  [unwired: 3 in]
  n94 = Number To Fractional String(number=w131) -> (F-format string=w105:string)  [unwired: 3 in]
  n95 = Number To Fractional String(number=w130) -> (F-format string=w104:string)  [unwired: 3 in]
  n96 = Number To Fractional String(number=w129) -> (F-format string=w103:string)  [unwired: 3 in]
  n97 = Number To Fractional String(number=w128) -> (F-format string=w102:string)  [unwired: 3 in]
  n98 = Number To Fractional String(number=w127) -> (F-format string=w101:string)  [unwired: 3 in]
  n99 = Number To Fractional String(number=w126) -> (F-format string=w100:string)  [unwired: 3 in]
  n100 = Number To Fractional String(number=w125) -> (F-format string=w99:string)  [unwired: 3 in]
  n101 = Number To Fractional String(number=w124) -> (F-format string=w98:string)  [unwired: 3 in]
  n102 = Number To Fractional String(number=w123) -> (F-format string=w97:string)  [unwired: 3 in]
  n103 = case shown="\"GEA Inlet Side Meter\", Default" w33 {
    tunnel: w60 -> [w208 w212]
    tunnel: [w201 w210] -> w58
    tunnel: w34 -> [w204 _]
    frame "GEA Inlet Side Meter", Default {
      n104 = Build Array (concatenate)("Hot Draw Amounts (gal)", w204, "" ("Numeric")) -> (w203:string[])
      n105 = Build Array (concatenate)("Cold Draw Amounts (gal)", w208, "" ("Numeric")) -> (w202:string[])
      n106 = Build Array(w203, w202) -> (w201:string[][])
    }
    frame "GEA Outlet Side Meter" {
      # "Outlet side meter is noted\nas the cold water"
      n107 = Build Array (concatenate)("Hot Draw Amounts (gal)", w212, "" ("Numeric")) -> (w211:string[])
      n108 = Build Array(w211) -> (w210:string[][])
    }
  }
  n109 = Build Array (concatenate)("Avg. Temperature Delivered (F)", w54, "" ("Numeric")) -> (w39:string[])
  n110 = Build Array (concatenate)("Hot Water Density (lb/gal)", w53, "" ("Numeric")) -> (w38:string[])
  n111 = Build Array (concatenate)("Cp Hot Water (BTU/(lbm F))", w52, "" ("Numeric")) -> (w37:string[])
  n112 = Build Array (concatenate)("Avg. Temperature Inlet (F)", w51, "" ("Numeric")) -> (w36:string[])
  n113 = Build Array (concatenate)("Cold Water Density (lb/gal)", w50, "" ("Numeric")) -> (w11:string[])
  n114 = Build Array (concatenate)("Max Flow Rate (GPM)", w21, "" ("Numeric")) -> (w18:string[])
  n115 = Build Array (concatenate)("Min Flow Rate (GPM)", w20, "" ("Numeric")) -> (w17:string[])
  n116 = Build Array (concatenate)("Max. Temperature Inlet (F)", w28, "" ("Numeric")) -> (w12:string[])
  n117 = Build Array (concatenate)("Min. Temperature Inlet (F)", w27, "" ("Numeric")) -> (w13:string[])
  n118 = Build Array (concatenate)("Draw Amounts (lbs)", w59, "" ("Numeric")) -> (w57:string[])
  n119 = Build Array (concatenate)("Draw Cluster Amounts (gal)", w55, "" ("Numeric")) -> (w40:string[])
  n120 = Build Array(w185, w184, w183, w182, w181, w180, w179, w178, w177, w176, w175, w174, w173, w172, w171, w122, w121, w120, w119, w118, w117, w116, w115, w114, w113, w112, w111, w110, w109, w108, w107, w106, w105, w104, w103, w102, w101, w100, w99, w98, w97) -> (w155:string[])
  n121 = Build Array(w68, w155) -> (w154:string[][])
  n122 = Transpose 2D Array(2D array=w154) -> (transposed array=w151:string[][])
  n123 = Build Array (concatenate)(w67, string[] [] ("array"), w151) -> (w150:string[][])
  n124 = Build Array (concatenate)(w58, w57, w40, w18, w17, w39, w38, w37, w36, w11, w12, w13) -> (w56:string[][])
  n125 = Transpose 2D Array(2D array=w56) -> (transposed array=w5:string[][])
  n126 = Build Array (concatenate)(w150, string[] [] ("array"), w5) -> (w65:string[][])
  n127 = Bundle By Name(cluster="UEF Calculated Values Output in", "Test Information.UEF Report Information"=w65) -> (→"UEF Calculated Values Output out":T1)
  "error out" <- "error in (no error)"
